vi "USB2XXX_LINEX_SlaveTest.vi"() -> ()   [LabVIEW 2010]
panel:
  in  "stop":bool
  out "从机读取到的数据帧数":i32
  in  "pInMsg 3":T1={"Timestamp"=20, "MsgType"=3, "CheckType"=1, "DataLen"=8, "Sync"=85, "PID"=3, "Data[0]"=33, "Data[1]"=34, "Data[2]"=35, "Data[3]"=36, "Data[4]"=37, "Data[5]"=38, "Data[6]"=39, "Data[7]"=40, "Check"=1, "Reserve"=0, "Reserve"=0} {"Sync" format="%x"; "PID" format="%x"; "Data[0]" format="%x"; "Data[1]" format="%x"; "Data[2]" format="%x"; "Data[3]" format="%x"; "Data[4]" format="%x"; "Data[5]" format="%x"; "Data[6]" format="%x"; "Data[7]" format="%x"; "Check" format="%x"; "Reserve" format="%x"; "Reserve" format="%x"}
  in  "pInMsg 2":T1={"Timestamp"=20, "MsgType"=3, "CheckType"=1, "DataLen"=8, "Sync"=85, "PID"=2, "Data[0]"=17, "Data[1]"=18, "Data[2]"=19, "Data[3]"=20, "Data[4]"=21, "Data[5]"=22, "Data[6]"=23, "Data[7]"=24, "Check"=1, "Reserve"=0, "Reserve"=0} {"Sync" format="%x"; "PID" format="%x"; "Data[0]" format="%x"; "Data[1]" format="%x"; "Data[2]" format="%x"; "Data[3]" format="%x"; "Data[4]" format="%x"; "Data[5]" format="%x"; "Data[6]" format="%x"; "Data[7]" format="%x"; "Check" format="%x"; "Reserve" format="%x"; "Reserve" format="%x"}
  out "pOutMsg":T2(array[cluster]) {"Sync" format="%x"; "PID" format="%x"; "Data[0]" format="%x"; "Data[1]" format="%x"; "Data[2]" format="%x"; "Data[3]" format="%x"; "Data[4]" format="%x"; "Data[5]" format="%x"; "Data[6]" format="%x"; "Data[7]" format="%x"; "Check" format="%x"}
  in  "pInMsg":T1={"Timestamp"=20, "MsgType"=3, "CheckType"=1, "DataLen"=8, "Sync"=85, "PID"=1, "Data[0]"=1, "Data[1]"=2, "Data[2]"=3, "Data[3]"=4, "Data[4]"=5, "Data[5]"=6, "Data[6]"=7, "Data[7]"=8, "Check"=1, "Reserve"=0, "Reserve"=0} {"Sync" format="%x"; "PID" format="%x"; "Data[0]" format="%x"; "Data[1]" format="%x"; "Data[2]" format="%x"; "Data[3]" format="%x"; "Data[4]" format="%x"; "Data[5]" format="%x"; "Data[6]" format="%x"; "Data[7]" format="%x"; "Check" format="%x"; "Reserve" format="%x"; "Reserve" format="%x"}
  out "function return":i32
  in  "BaudRate":u32=19200
  in  "Channel Index":u8(ring) items=["LIN1", "LIN2"]
  in  "Device Index":i32(ring) items=["0", "1", "2", "3", "4", "5"]
  # "波特率一定要设置，否则程序可能出错"
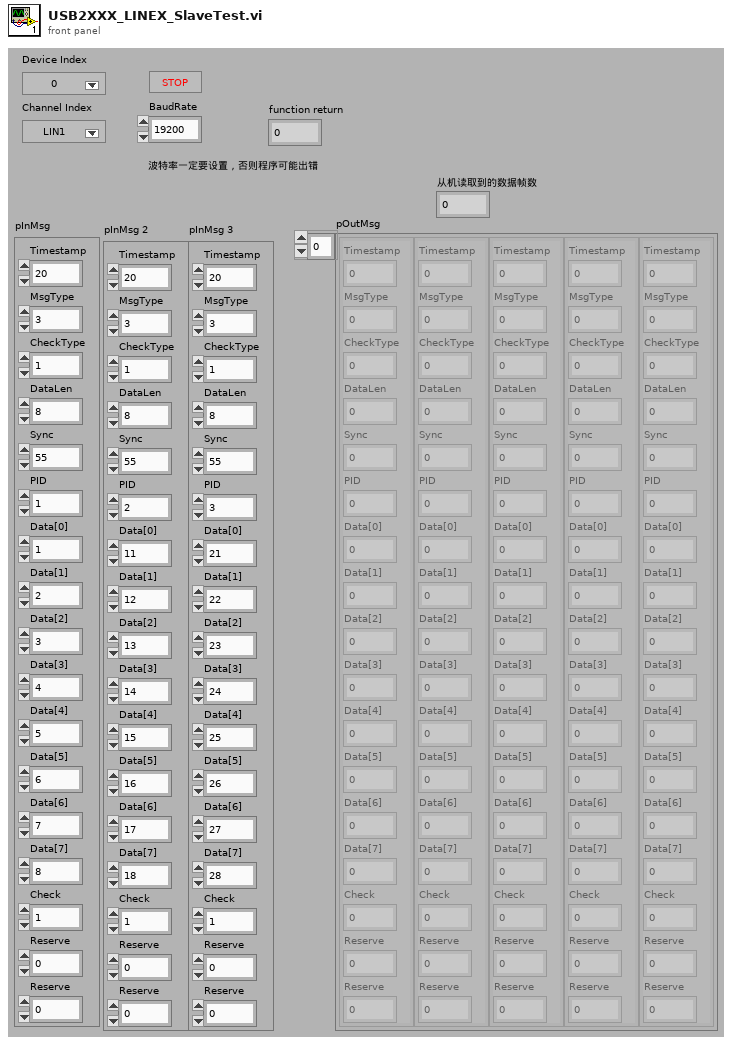
[diagram p1: front panel]
types:
  T1 = cluster{"Timestamp":u32, "MsgType":u8, "CheckType":u8, "DataLen":u8, "Sync":u8, "PID":u8, "Data[0]":u8, "Data[1]":u8, "Data[2]":u8, "Data[3]":u8, "Data[4]":u8, "Data[5]":u8, "Data[6]":u8, "Data[7]":u8, "Check":u8, "Reserve":u8, "Reserve":u8}
  T2 = cluster{"Timestamp":u32, "MsgType":u8, "CheckType":u8, "DataLen":u8, "Sync":u8, "PID":u8, "Data[0]":u8, "Data[1]":u8, "Data[2]":u8, "Data[3]":u8, "Data[4]":u8, "Data[5]":u8, "Data[6]":u8, "Data[7]":u8, "Check":u8, "Reserve":u8, "Reserve":u8}[]
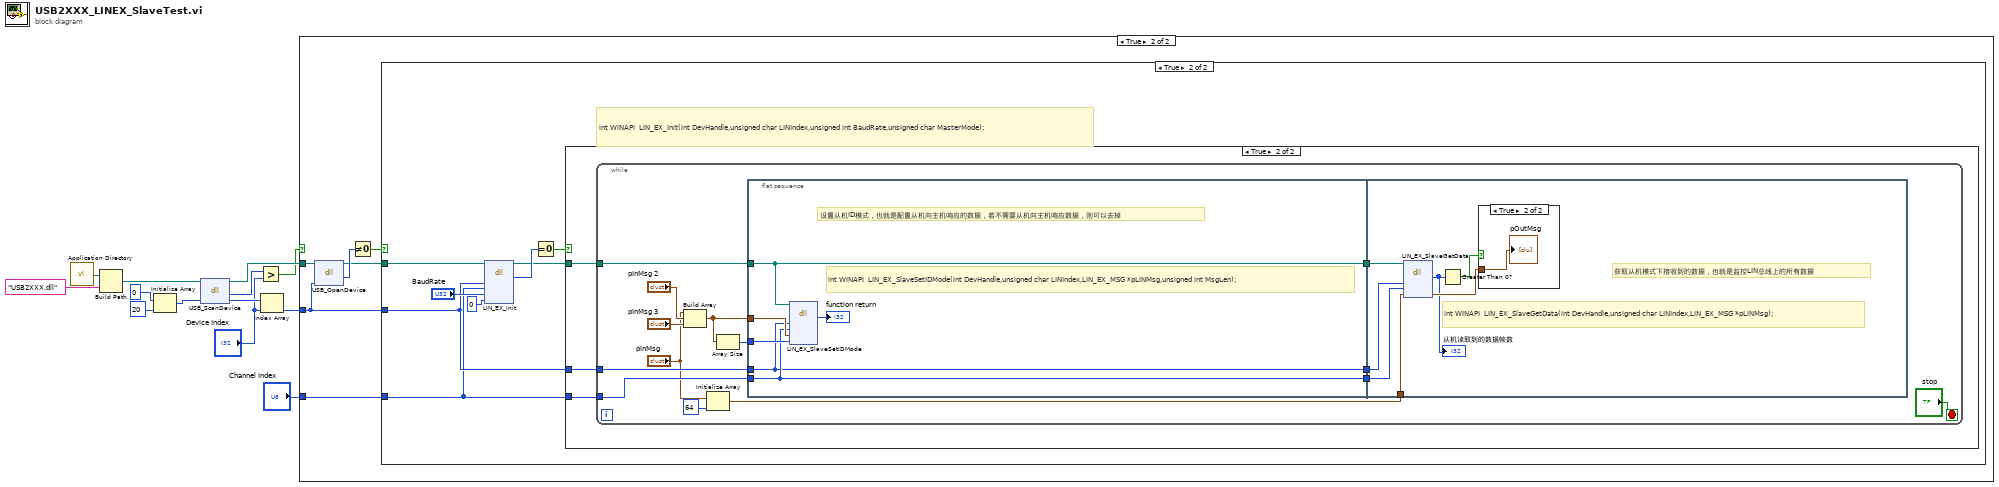
[diagram p0: block diagram]
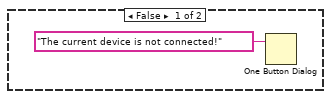
[diagram p2: hidden frame]
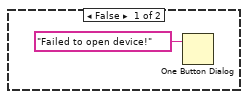
[diagram p3: hidden frame]
diagram:
  n1 = call <vilib>:"Application Directory.vi"() -> ("Application Directory"=w6:path)
  n2 = Build Path(base path=w6, name or relative path="USB2XXX.dll") -> (appended path=w5:path)
  n3 = Initialize Array(0, 20 ("dimension size")) -> (w10:i32[])
  n4 = dll-call lib="E:/OtherWork/STM32/USB2XXX_Example/trunk/Labview/PublicFiles/USB2XXX.dll" fn="USB_ScanDevice"(path in=w5, "pDevNum"=w10) -> (path out=w8:path, "return type"=w3:i32, "pDevNum"=w13:i32[])  [unwired: 2 in, 1 out]
  n5 = Greater?(x=w3, y="Device Index") -> (0:w4:bool)
  n6 = Index Array(array=w13, index="Device Index") -> (element=w9:i32)
  n7 = case shown="True" w4 {
    tunnel: w9 -> [_ w16]
    tunnel: w8 -> [_ w19]
    tunnel: "Channel Index" -> [_ w15]
    frame False {
      n8 = One Button Dialog(message="The current device is not connected!") -> ()  [unwired: 1 in, 1 out]
    }
    frame True {
      n9 = dll-call lib="E:/OtherWork/STM32/USB2XXX_Example/trunk/Labview/PublicFiles/USB2XXX.dll" fn="USB_OpenDevice"(path in=w19, "DevIndex"=w16) -> (path out=w17:path, "return type"=w20:u8)  [unwired: 3 in, 1 out]
      n10 = Not Equal To 0?(x=w20) -> (x != 0?=w18:bool)
      n11 = case shown="True" w18 {
        tunnel: w17 -> [_ w27]
        tunnel: w16 -> [_ w24]
        tunnel: w15 -> [_ w23]
        frame False {
          n12 = One Button Dialog(message="Failed to open device!") -> ()  [unwired: 1 in, 1 out]
        }
        frame True {
          # "int WINAPI  LIN_EX_Init(int DevHandle,unsigned char LINIndex,unsigned int BaudRate,unsigned char MasterMode);"
          n13 = dll-call lib="E:/OtherWork/STM32/USB2XXX_Example/trunk/Labview/PublicFiles/USB2XXX.dll" fn="LIN_EX_Init"(path in=w27, "DevHandle"=w24, "LINIndex"=w23, "BaudRate"="BaudRate", "MasterMode"=u8 0) -> (path out=w22:path, "return type"=w26:i32)  [unwired: 6 in, 1 out]
          n14 = Equal To 0?(x=w26) -> (x = 0?=w25:bool)
          n15 = case shown="True" w25 {
            tunnel: w24 -> [_ w32]
            tunnel: w23 -> [_ w31]
            tunnel: w22 -> [_ w30]
            frame False {
            }
            frame True {
              n16 = while {
                tunnel: w32 -> [w41]
                tunnel: w31 -> [w40]
                tunnel: w30 -> [w37]
                stop <- "stop" stop-if-true
                n17 = Build Array("pInMsg", "pInMsg 2", "pInMsg 3") -> (w39:T2)
                n18 = Initialize Array("pInMsg", 64 ("dimension size")) -> (w34:T2)
                n19 = Array Size(array=w39) -> (size(s)=w38:i32)
                n20 = flat-sequence {
                  tunnel: w41 -> [w48]
                  tunnel: w40 -> [w49]
                  tunnel: w39 -> [w52]
                  tunnel: w38 -> [w51]
                  tunnel: w37 -> [w47]
                  tunnel: [w49] -> w46
                  tunnel: [w48] -> w45
                  tunnel: [w47] -> w44
                  tunnel: w34 -> [w59]
                  tunnel: w46 -> [w58]
                  tunnel: w45 -> [w57]
                  tunnel: w44 -> [w56]
                  frame #0 {
                    # "设置从机ID模式，也就是配置从机向主机响应的数据，若不需要从机向主机响应数据，则可以去掉"
                    # "int WINAPI  LIN_EX_SlaveSetIDMode(int DevHandle,unsigned char LINIndex,LIN_EX_MSG *pLINMsg,unsigned int MsgLen);"
                    n21 = dll-call lib="E:/OtherWork/STM32/USB2XXX_Example/trunk/Labview/PublicFiles/USB2XXX.*" fn="LIN_EX_SlaveSetIDMode"(path in=w47, "DevHandle"=w48, "LINIndex"=w49, "pLINMsg"=w52, "MsgLen"=w51) -> ("return type"=→"function return":i32)  [unwired: 6 in, 2 out]
                  }
                  frame #1 {
                    # "获取从机模式下接收到的数据，也就是监控LIN总线上的所有数据"
                    # "int WINAPI  LIN_EX_SlaveGetData(int DevHandle,unsigned char LINIndex,LIN_EX_MSG *pLINMsg);"
                    n22 = dll-call lib="E:/OtherWork/STM32/USB2XXX_Example/trunk/Labview/PublicFiles/USB2XXX.*" fn="LIN_EX_SlaveGetData"(path in=w56, "DevHandle"=w57, "LINIndex"=w58, "pLINMsg"=w59) -> ("return type"=w54:i32, "pLINMsg"=w55:T2)  [unwired: 4 in, 2 out]
                    "从机读取到的数据帧数" <- w54
                    n23 = Greater Than 0?(x=w54) -> (x > 0?=w53:bool)
                    n24 = case shown="True" w53 {
                      tunnel: w55 -> [_ w60]
                      frame False {
                      }
                      frame True {
                        "pOutMsg" <- w60
                      }
                    }
                  }
                }
              }
            }
          }
        }
      }
    }
  }
